vi "Get Desired Size.vi"(8 "error in (no error)":errorcluster, 11 "ColorArrayPanel in":refnum<class "ColorArrayPanel.lvclass">) -> (0 "error out":errorcluster, 2 "Desired Size":T1, 3 "ColorArrayPanel out":refnum<class "ColorArrayPanel.lvclass">)   [LabVIEW 2020, in "Nested.lvlib" / "ColorArrayPanel.lvclass"]
uses:
  ColorArrayPanel.lvclass
  OOPanel/Desired Size.ctl
  OOPanel/OOPanel.lvlib
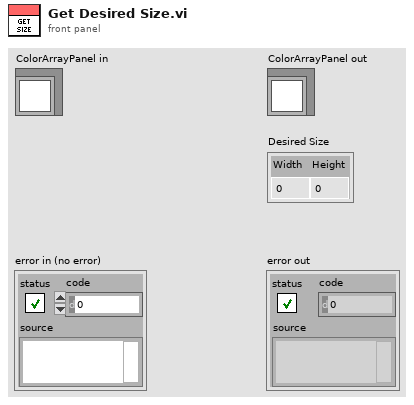
[diagram p1: front panel]
types:
  T1 = typedef "OOPanel.lvlib/Desired Size.ctl" = cluster{"Width":u32, "Height":u32}
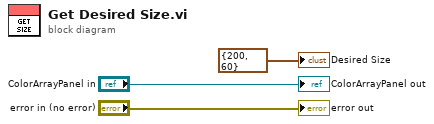
[diagram p0: block diagram]
diagram:
  "error out" <- "error in (no error)"
  "ColorArrayPanel out" <- "ColorArrayPanel in"
  "Desired Size" <- T1 {"Width"=200, "Height"=60} ("Desired Size")
